vi "Set Resource Purpose.vi"(10 "Resource Purpose":string, 11 "Resource in":refnum<class "Resource.lvclass">) -> (3 "Resource out":refnum<class "Resource.lvclass">)   [LabVIEW 2020]
uses:
  Resource.lvclass/Resource.ctl
  Resource.lvclass
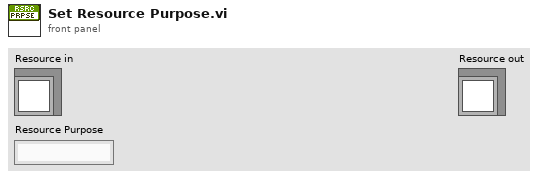
[diagram p1: front panel]
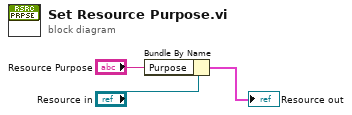
[diagram p0: block diagram]
diagram:
  n1 = Bundle By Name(cluster="Resource in", "Purpose"="Resource Purpose") -> (→"Resource out":cluster{})
